vi "MSP6715-Link.vi"(8 "error in":errorcluster caption="错误输入（无错误）", 10 "等待时间(毫秒)":u32=100, 11 "MyIndex":u8) -> (0 "error out":errorcluster)   [LabVIEW 2015, in "MSP6715.lvlib"]
uses:
  MSP6715.lvlib
  <vilib>/Instr/_visa.llb/VISA Configure Serial Port (Instr).vi
panel:
  out "返回值":u8[](array[numeric])
  out "VISA":refnum<visa-resource-name>
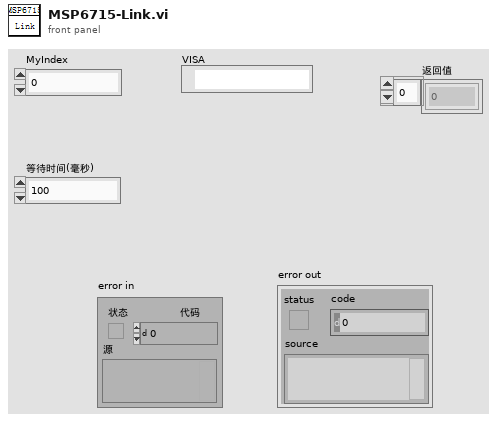
[diagram p1: front panel]
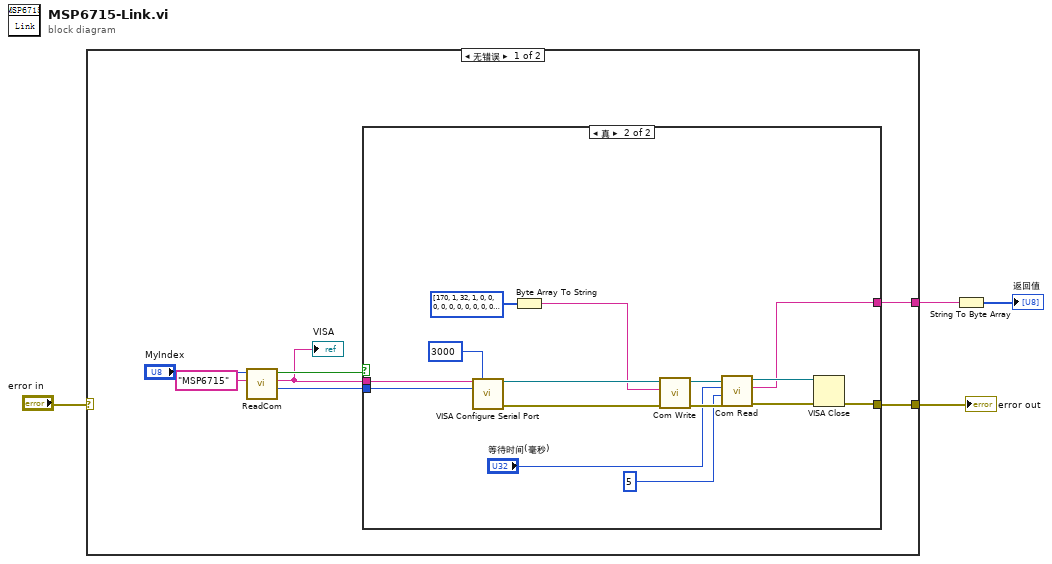
[diagram p0: block diagram]
diagram:
  n1 = case shown="无错误" "error in" {
    selector: "error in" -> [_ w27]
    tunnel: [w11 w27] -> w4
    tunnel: [w5 _] -> w2
    frame No Error {
      n2 = call "ReadCom.vi"("仪器名称"="MSP6715", "MyIndex"="MyIndex") -> ("Baudrate"=w6:i32, "COM"=w7:string, "OK?"=w8:bool)  [unwired: 7 in]
      "VISA" <- w7
      n3 = case shown="真" w8 {
        tunnel: [_ w26] -> w11
        tunnel: w7 -> [_ w25]
        tunnel: w6 -> [_ w24]
        tunnel: [_ w16] -> w5
        frame False {
        }
        frame True {
          n4 = call-poly "VISA Configure Serial Port"("VISA resource name"=w25, "timeout (10sec)"=u32 3000, "baud rate (9600)"=w24) -> ("VISA resource name out"=w22:refnum<visa-resource-name>, "error out"=w21:errorcluster)  [unwired: 11 in]
          n5 = Byte Array To String(unsigned byte array=u32[] [170, 1, 32, 1, 0, 0, 0, 0, 0, 0, 0, 0, 0, 0, 0, 0, 0, 0, 0, 0, 0, 0, 0, 0, 0, 204] ("Hex指令")) -> (string=w12:string)
          n6 = call "Com Write.vi"("错误输入（无错误）"=w21, "Wbuff"=w12, "VISA In"=w22) -> ("错误输出"=w19:errorcluster, "VISA Out"=w20:refnum<visa-resource-name>)  [unwired: 7 in]
          n7 = call "Com Read.vi"("错误输入（无错误）"=w19, "num"=u32 5, "超时"="等待时间(毫秒)", "VISA In"=w20) -> ("错误输出"=w18:errorcluster, "buff"=w16:string, "VISA Out"=w17:refnum<visa-resource-name>)  [unwired: 5 in]
          n8 = VISA Close(VISA resource name=w17, error in (no error)=w18) -> (error out=w26:errorcluster)
        }
      }
    }
    frame Error {
    }
  }
  "error out" <- w4
  n9 = String To Byte Array(string=w2) -> (unsigned byte array=→"返回值":u8[])
